vi "global variables.vi"() -> ()   [LabVIEW 2017]
uses:
  Classes/StatusLog/StatusLog.lvclass
  Classes/Message/Message.lvclass
  Classes/PrepLineObject/PrepLineObject.lvclass
  Classes/Flags/flag.lvclass
  Classes/Plots/Plots.lvclass
  Classes/Standard/Standard.lvclass
  Classes/Spectrometer/Spectrometer.lvclass
  Classes/Analysis/Analysis.lvclass
  Classes/Instrument/instrument.lvclass
  Classes/MagFieldTable/MagFieldTable.lvclass
  Classes/Pipette/Pipette.lvclass
panel:
  in  "PipObjects":refnum<queue>
  in  "RunScriptsFolder":path
  out "MFTObjQueue":refnum<queue>
  out "InstrObjQueue":refnum<queue>
  out "AnalysisObjQueue":refnum<queue>
  in  "results folder":path
  in  "SpecObjQueue":refnum<queue>
  in  "StdObjQueue":refnum<queue>
  in  "user event out":refnum<user-event>
  in  "PlotObjQueue":refnum<queue>
  in  "FlagObjQueue":refnum<queue>
  out "PrepLineObjQueue":refnum<queue>
  out "SysChkBuffer":u32=1000
  in  "ScriptMsgObj":refnum<class "Message.lvclass">
  in  "LogFileObj":refnum<class "StatusLog.lvclass">
  out "SysChkIntervall":u32=60000
  in  "close prog flag":bool
  # "Object References"
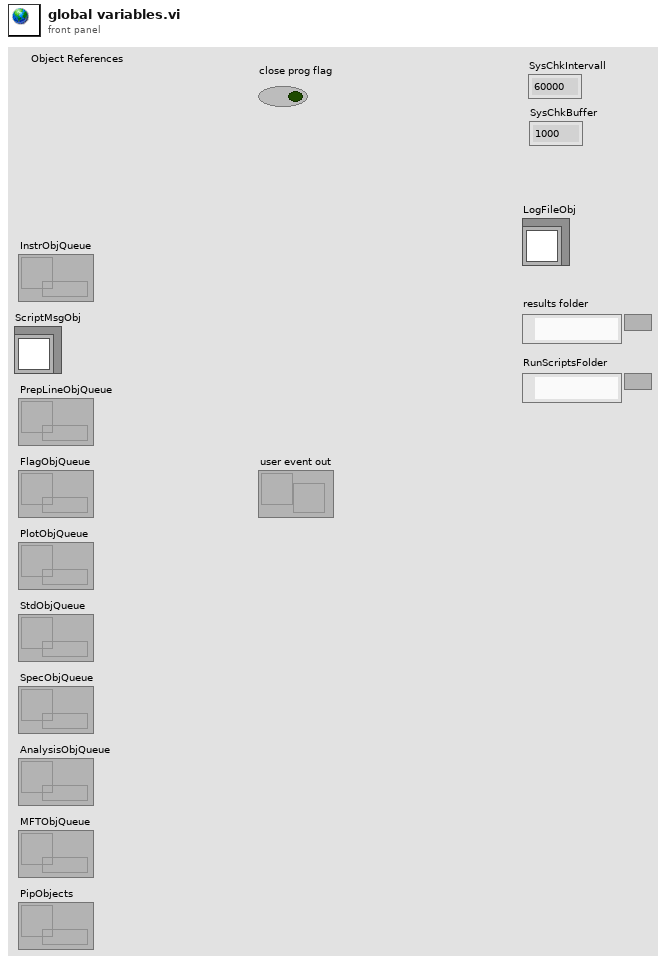
[diagram p1: front panel]
diagram:
